vi "terminate.vi"(8 "error in (no error)":errorcluster, 11 "GenericPlugin in":refnum<class "FPGAWrapperDL090211Galvo_grabber.lvclass">) -> (0 "error out":errorcluster, 3 "GenericPlugin out":refnum<class "FPGAWrapperDL090211Galvo_grabber.lvclass">)   [LabVIEW 2010, in "FPGAWrapperDL090211Galvo_grabber.lvclass"]
doc: "The dynamic dispatch version of this VI terminates the plug-in object by releasing all of its resources."
uses:
  FPGAWrapperDL090211Galvo_grabber.lvclass
  FPGAWrapperDL090211Galvo_grabber.lvclass/FPGAWrapperDL090211Galvo_grabber.ctl
  type definitions/command_enum.ctl
  GenericFPGAWrapper/GenericFPGAWrapper/GenericFPGAWrapper.lvclass
  class_data.vi
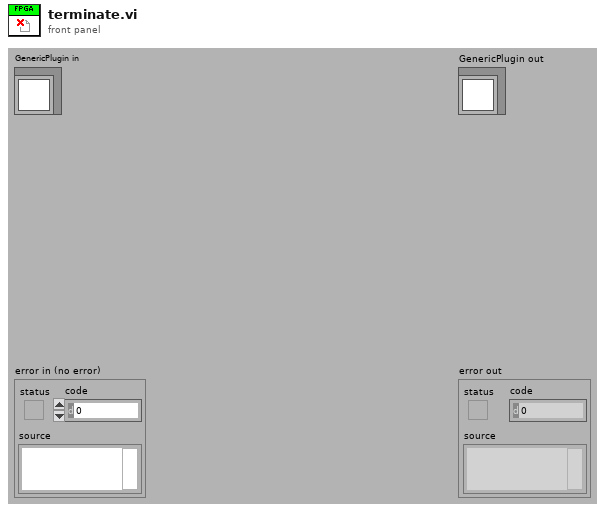
[diagram p1: front panel]
types:
  T1 = typedef "command_enum.ctl" = enum16{"NULL", "update", "start", "stop", "reset", "shut-down"}
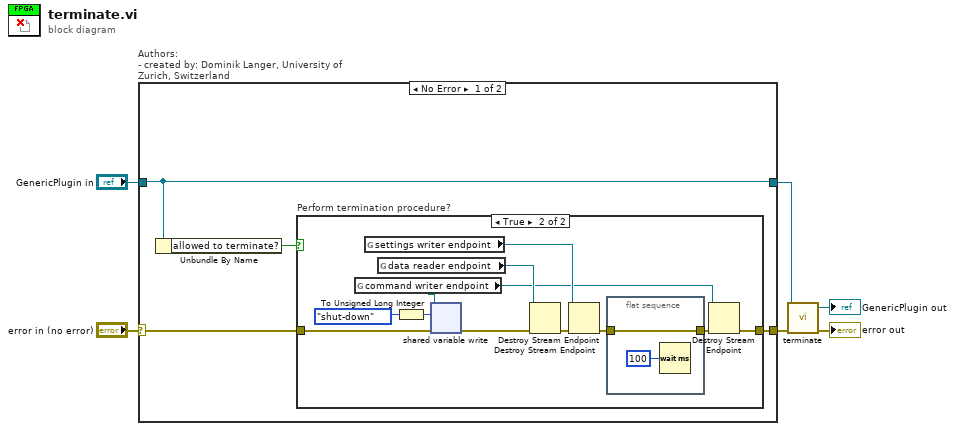
[diagram p0: block diagram]
diagram:
  n1 = case "Authors: \n- created by: Dominik Langer, University of Zurich, Switzerland" shown="No Error" "error in (no error)" {
    selector: "error in (no error)" -> [w10 w26]
    tunnel: "GenericPlugin in" -> [w8 w25]
    tunnel: [w9 w26] -> w2
    tunnel: [w8 w25] -> w1
    frame No Error {
      n2 = Unbundle By Name(w8) -> ("allowed to terminate?"=w7:bool)
      n3 = case "Perform termination procedure?" shown="True" w7 {
        tunnel: w10 -> [w11 w20]
        tunnel: [w11 w16] -> w9
        frame False {
        }
        frame True {
          n4 = global read "class_data.vi" "command writer endpoint"() -> (w14:refnum<k21>)
          n5 = global read "class_data.vi" "settings writer endpoint"() -> (w15:refnum<k21>)
          n6 = global read "class_data.vi" "data reader endpoint"() -> (w18:refnum<k21>)
          n7 = To Unsigned Long Integer(number=command_enum."shut-down" ("command")) -> (unsigned 32bit integer=w22:u32)
          n8 = shared-variable-write(w14, w20, w22) -> (w19:errorcluster)  [unwired: 1 in, 2 out]
          n9 = Destroy Stream Endpoint(8:w19, 11:w18) -> (0:w17:errorcluster)
          n10 = Destroy Stream Endpoint(8:w17, 11:w15) -> (0:w13:errorcluster)
          n11 = flat-sequence {
            tunnel: [w24] -> w12
            tunnel: w13 -> [w24]
            frame #0 {
              n12 = Wait (ms)(milliseconds to wait=u32 100) -> ()  [unwired: 1 out]
            }
          }
          n13 = Destroy Stream Endpoint(8:w12, 11:w14) -> (0:w16:errorcluster)
        }
      }
    }
    frame Error {
    }
  }
  n14 = call-parent "terminate.vi"("error in (no error)"=w2, "GenericPlugin in"=w1) -> ("error out"=→"error out":errorcluster, "GenericPlugin out"=→"GenericPlugin out":refnum<class "FPGAWrapperDL090211Galvo_grabber.lvclass">)  [unwired: 8 in]
